vi "02_ui_smith_plot.vi"() -> ()   [LabVIEW 2025]
uses:
  213d4d69-42c2-4ab9-8e5c-f09799411473.vi
  9924c898-3be5-4834-b900-de0bc968c1de.vi
  9ab8033c-be5d-4a17-bbd5-1ebfae571c10.vi
panel:
  out "r_norm":dbl caption="Cursor - R"
  out "jx_norm":dbl caption="Cursor - jX"
  out "phase_cursor":dbl caption="Phase"
  out "jx_cursor":dbl caption="jX"
  out "r_cursor":dbl caption="R"
  out "smith_dimensions":i16
  out "frequency_cursor":string caption="Frequency"
  out "panel_resized":bool=TRUE
  out "smith_plot":picture
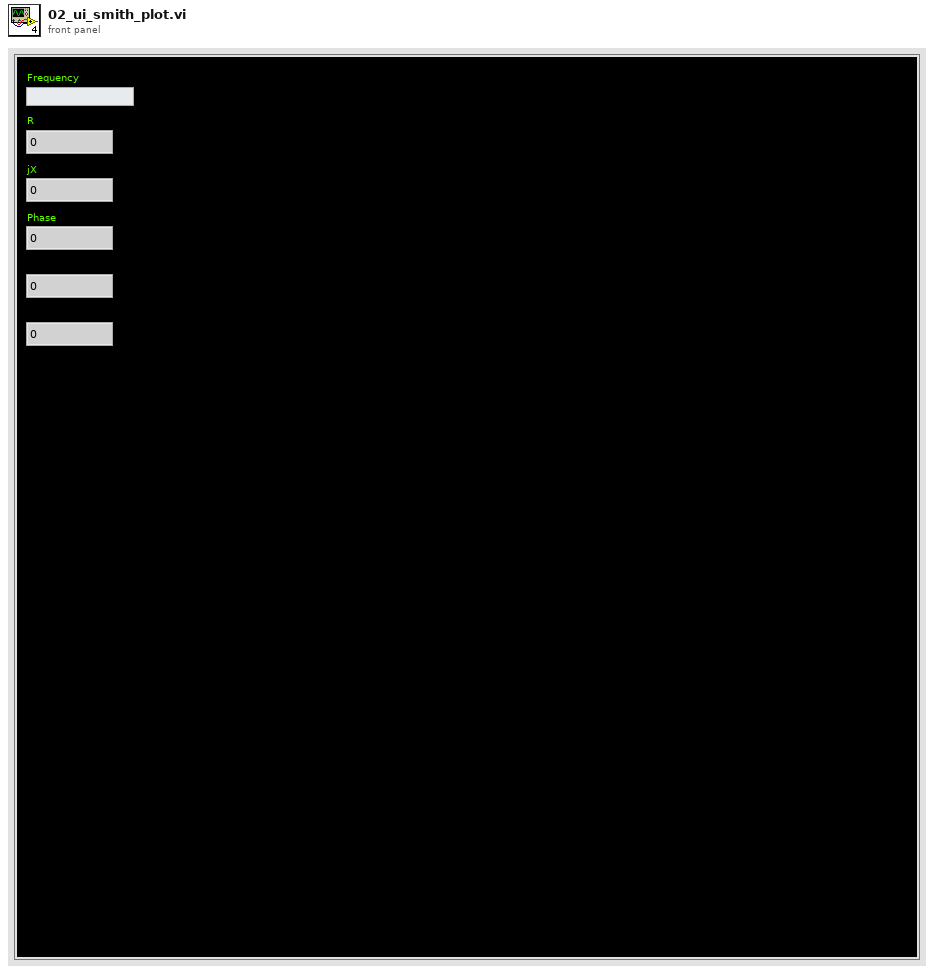
[diagram p1: front panel]
types:
  T1 = cluster{"button_load_sxp":bool, "button_load_csv":bool, "button_save_s1p":bool, "button_save_s2p":bool, "button_single_sweep":bool, "show_smith_window":bool}
  T2 = cluster{"freq_array":dbl[], "data_array":dbl[]}[]
  T3 = typedef "LVRectTypeDef.ctl" = cluster{"Left":i16, "Top":i16, "Right":i16, "Bottom":i16}
  T4 = typedef "LVPoint32TypeDef.ctl" = cluster{"Horizontal":i32, "Vertical":i32}
  T5 = cluster{"frequency":dbl, "r":dbl, "jx":dbl, "phase":dbl}
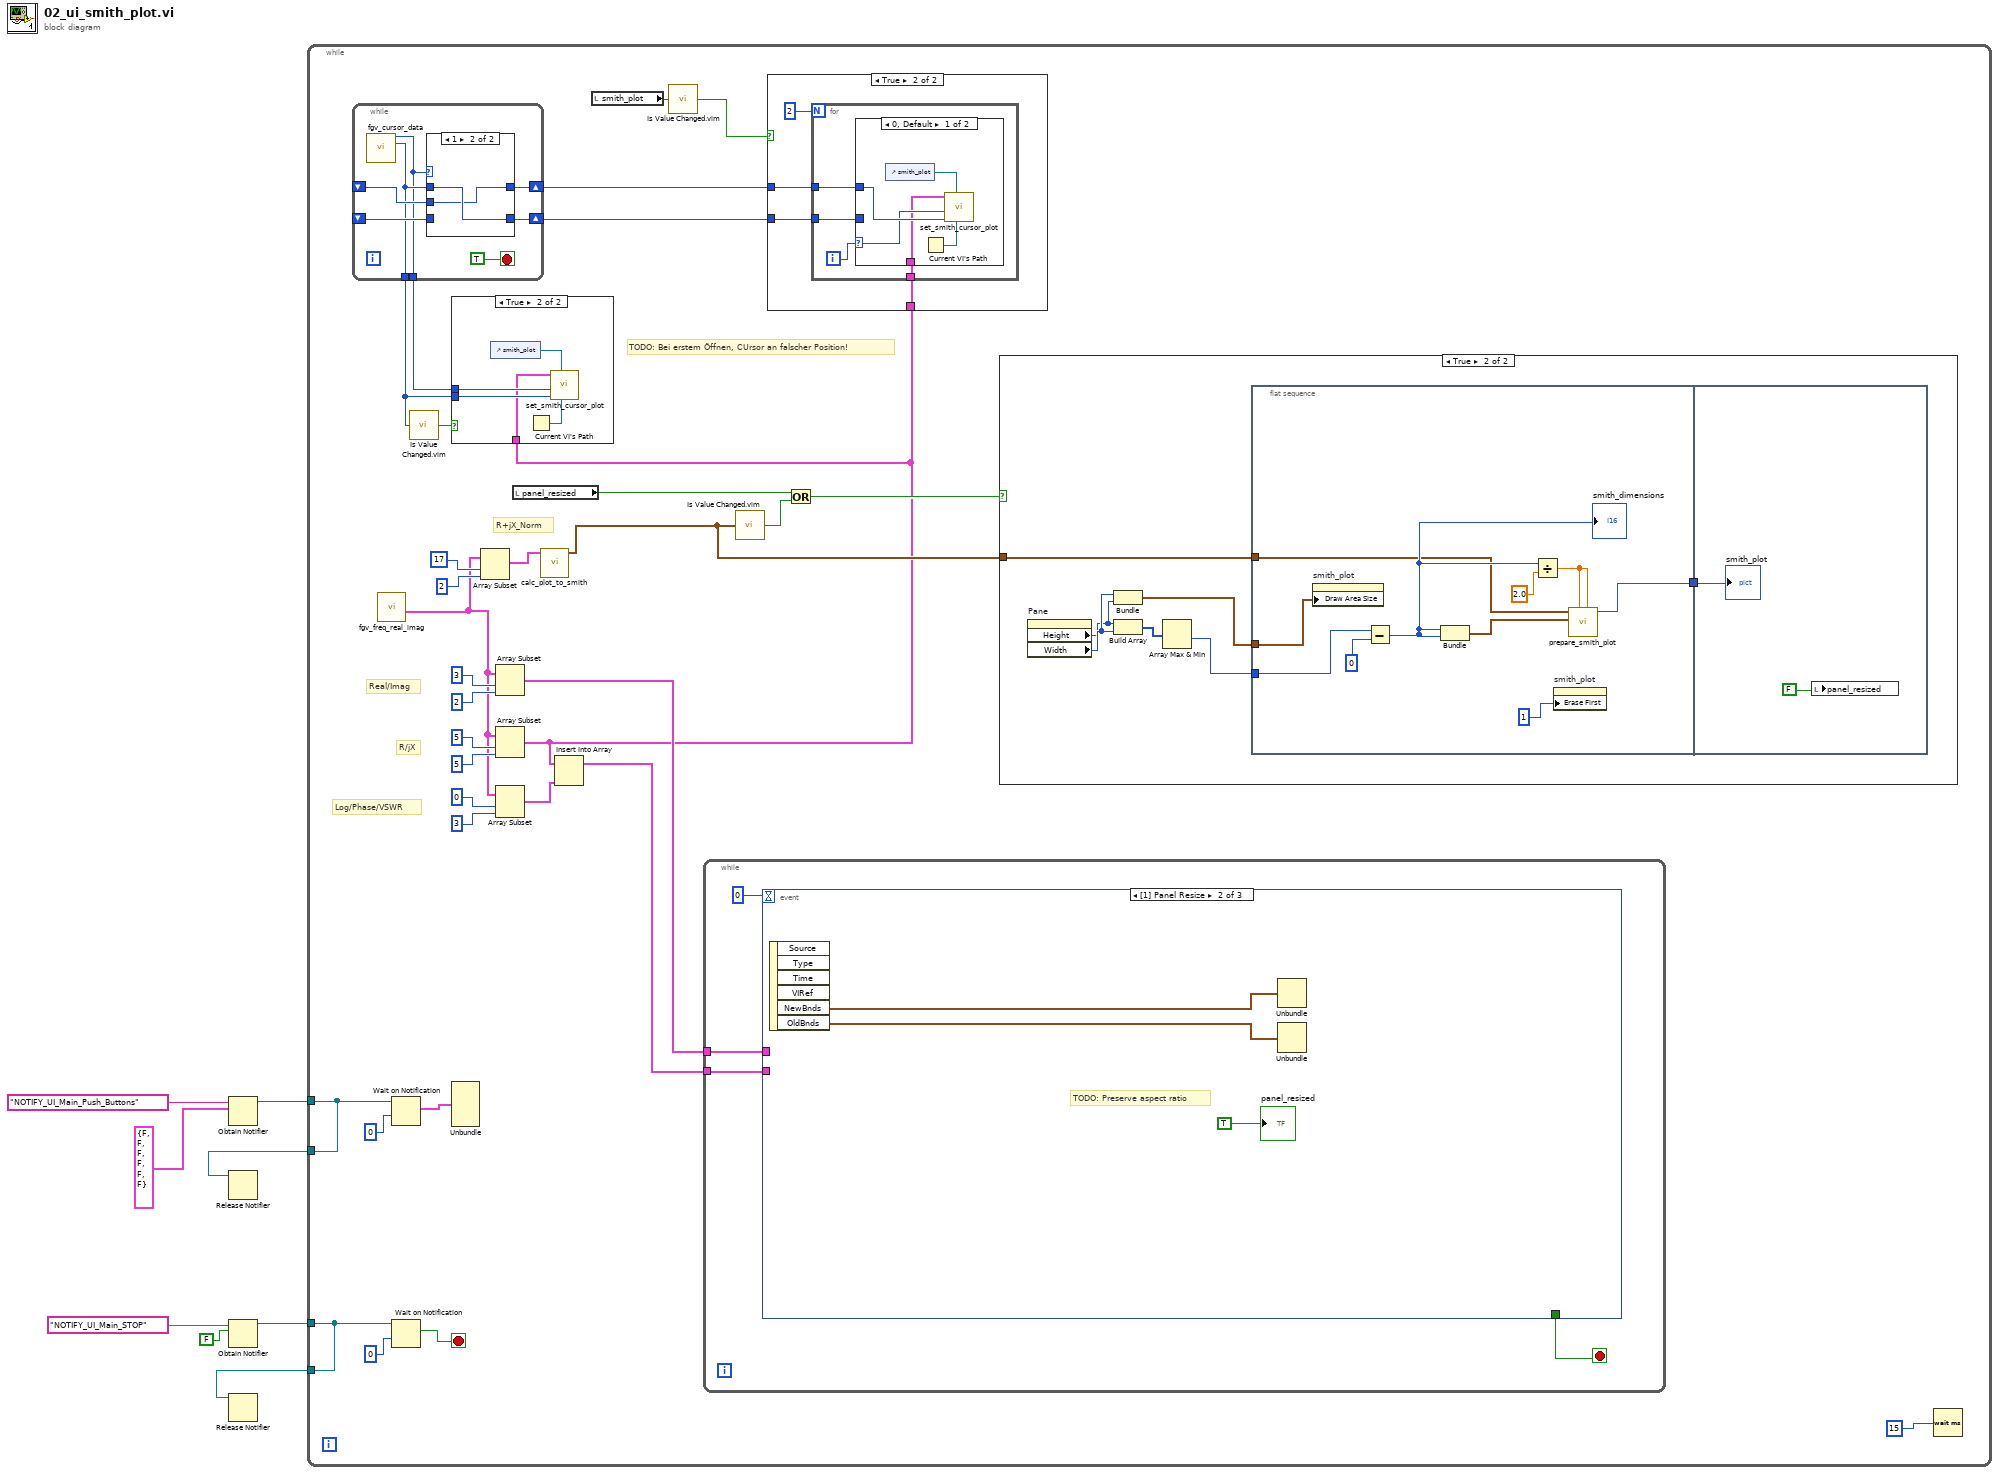
[diagram p0: block diagram]
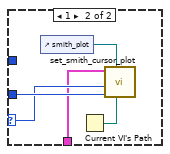
[diagram p4: hidden frame]
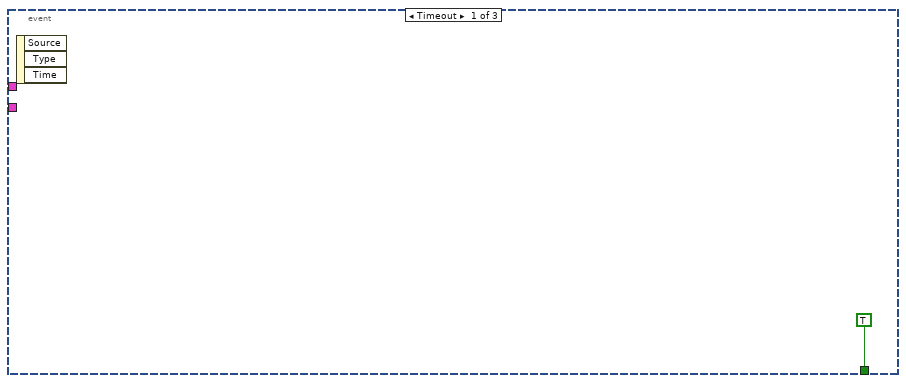
[diagram p6: hidden frame]
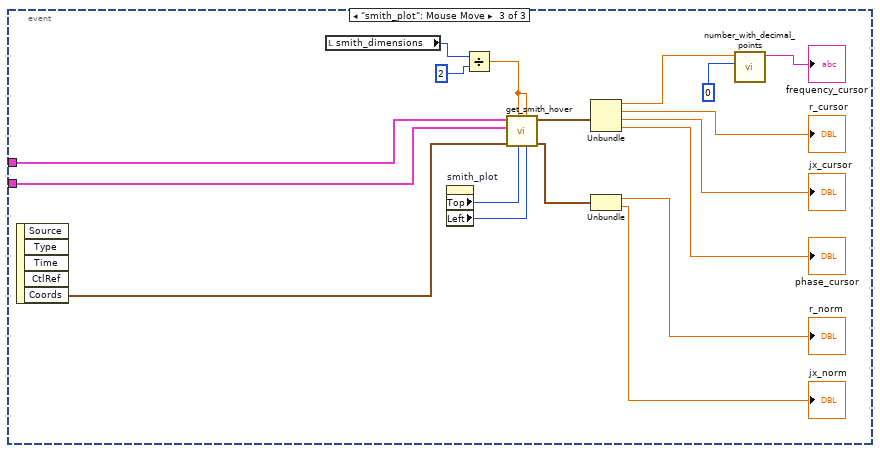
[diagram p7: hidden frame]
diagram:
  n1 = Obtain Notifier(name (unnamed)="NOTIFY_UI_Main_Push_Buttons", notification data type=T1 {"button_load_sxp"=FALSE, "button_load_csv"=FALSE, "button_save_s1p"=FALSE, "button_save_s2p"=FALSE, "button_single_sweep"=FALSE, "show_smith_window"=FALSE} ("output cluster")) -> (notifier out=w2:refnum<notifier>)  [unwired: 2 in, 2 out]
  n2 = Obtain Notifier(name (unnamed)="NOTIFY_UI_Main_STOP", notification data type=FALSE) -> (notifier out=w6:refnum<notifier>)  [unwired: 2 in, 2 out]
  n3 = while {
    tunnel: w6 -> [w36]
    tunnel: [w36] -> w5
    tunnel: w2 -> [w29]
    tunnel: [w29] -> w1
    stop <- w35 stop-if-true
    # "TODO: Bei erstem Öffnen, CUrsor an falscher Position!"
    # "Log/Phase/VSWR"
    # "R/jX"
    # "Real/Imag"
    # "R+jX_Norm"
    n4 = while {
      shift-right: [w69] -> w16
      shift-left: _ -> [w67]
      shift-right: [w68] -> w17
      shift-left: _ -> [w66]
      tunnel: [w65] -> w12
      tunnel: [w64] -> w15
      stop <- TRUE stop-if-true
      n5 = call "fgv_cursor_data.vi"() -> ("cursor_idx_get"=w64:i32, "cursor_pos_get"=w65:i32)  [unwired: 9 in, 5 out]
      n6 = case shown="1" w64 {
        tunnel: w65 -> [w72 w74]
        tunnel: [w72 w73] -> w69
        tunnel: [w71 w74] -> w68
        tunnel: w67 -> [_ w73]
        tunnel: w66 -> [w71 _]
        frame 0, Default {
        }
        frame 1 {
        }
      }
    }
    n7 = call "fgv_freq_real_imag.vi"() -> ("plot_data"=w18:T2)  [unwired: 8 in, 3 out]
    n8 = Wait on Notification(notifier=w29, timeout in ms (-1)=0) -> (notification=w31:T1)  [unwired: 2 in, 3 out]
    n9 = Wait on Notification(notifier=w36, timeout in ms (-1)=0) -> (notification=w35:bool)  [unwired: 2 in, 3 out]
    n10 = call "Is Value Changed.vim"("value"=w12) -> ("changed or first call?"=w11:bool)
    n11 = Unbundle(w31) -> ()  [unwired: 6 out]
    n12 = Array Subset(array=w18, index=17, length=2) -> (w32:T2)
    n13 = Array Subset(array=w18, index=3, length=2) -> (w20:T2)
    n14 = Array Subset(array=w18, index=5, length=5) -> (w14:T2)
    n15 = case shown="True" w11 {
      tunnel: w12 -> [_ w43]
      tunnel: w15 -> [_ w42]
      tunnel: w14 -> [_ w41]
      frame False {
      }
      frame True {
        n16 = control-ref of="smith_plot"() -> (w44:refnum<vi>)
        n17 = Current VI's Path() -> (path=w45:path)
        n18 = call "set_smith_cursor_plot.vi"("path"=w45, "smith_plot"=w44, "cursor_pos"=w43, "cursor_index"=w42, "plot_rjx"=w41) -> ()  [unwired: 7 in]
      }
    }
    n19 = Array Subset(array=w18, index=0, length=3) -> (w22:T2)
    n20 = local read "panel_resized"() -> (w10:bool)
    n21 = call "calc_plot_to_smith.vi"("Plot_Data"=w32) -> ("smith plot"=w19:cluster{"r":dbl, "x":dbl}[])  [unwired: 10 in]
    n22 = Insert Into Array(array=w14, new element=w22) -> (w21:T2)  [unwired: 1 in]
    n23 = local read "smith_plot"() -> (w13:picture)
    n24 = call "Is Value Changed.vim"("value"=w13) -> ("changed or first call?"=w9:bool)
    n25 = while {
      tunnel: w21 -> [w76]
      tunnel: w20 -> [w75]
      stop <- w77 stop-if-true
      n26 = event shown="[1] Panel Resize" {
        selector: _ -> [_ _ _]
        dyn-events: _ -> [_ _ _]
        timeout: 0 -> [_ _ _]
        tunnel: [TRUE _ _] -> w77
        tunnel: w76 -> [_ _ w84]
        tunnel: w75 -> [_ _ w83]
        event Timeout {
          n27 = event-data() -> ()  [unwired: 1 in, 3 out]
        }
        event Panel Resize {
          # "TODO: Preserve aspect ratio"
          n28 = event-data() -> ("NewBnds"=w80:T3, "OldBnds"=w81:T3)  [unwired: 1 in, 4 out]
          n29 = Unbundle(w80) -> ()  [unwired: 4 out]
          n30 = Unbundle(w81) -> ()  [unwired: 4 out]
          "panel_resized" <- TRUE
        }
        event "smith_plot": Mouse Move {
          n31 = event-data() -> ("Coords"=w100:T4)  [unwired: 1 in, 4 out]
          n32 = local read "smith_dimensions"() -> (w95:i16)
          n33 = property on="smith_plot" class="Pict"() -> ("Top"=w98:i32, "Left"=w97:i32)  [unwired: 2 in, 2 out]
          n34 = Divide(x=w95, y=u32 2) -> (x/y=w93:dbl)
          n35 = call "get_smith_hover.vi"("smith_pos_left"=w97, "left_center"=w93, "smith_pos_top"=w98, "top_center"=w93, "Coords"=w100, "cursor_data"=w84, "ref_data"=w83) -> ("cursor_pos"=w87:cluster{"r_norm":dbl, "x_norm":dbl}, "cursor_data"=w92:T5)  [unwired: 3 in]
          n36 = Unbundle(w92) -> ("frequency"=w88:dbl, "r"=→"r_cursor":dbl, "jx"=→"jx_cursor":dbl, "phase"=→"phase_cursor":dbl)
          n37 = Unbundle(w87) -> ("r_norm"=→"r_norm":dbl, "x_norm"=→"jx_norm":dbl)
          n38 = call "number_with_decimal_points.vi"("Precision"=i16 0, "Double"=w88) -> ("String"=→"frequency_cursor":string)  [unwired: 5 in]
        }
      }
    }
    n39 = call "Is Value Changed.vim"("value"=w19) -> ("changed or first call?"=w38:bool)
    n40 = case shown="True" w9 {
      tunnel: w16 -> [_ w48]
      tunnel: w17 -> [_ w47]
      tunnel: w14 -> [_ w46]
      frame False {
      }
      frame True {
        n41 = for {
          N: 2 -> [_]
          tunnel: w48 -> [w52]
          tunnel: w47 -> [w51]
          tunnel: w46 -> [w50]
          i -> [w53]
          n42 = case shown="0, Default" w53 {
            selector: w53 -> [w55 w60]
            tunnel: w52 -> [w56 _]
            tunnel: w51 -> [_ w61]
            tunnel: w50 -> [w54 w59]
            frame 0, Default {
              n43 = control-ref of="smith_plot"() -> (w58:refnum<vi>)
              n44 = Current VI's Path() -> (path=w57:path)
              n45 = call "set_smith_cursor_plot.vi"("path"=w57, "smith_plot"=w58, "cursor_pos"=w56, "cursor_index"=w55, "plot_rjx"=w54) -> ()  [unwired: 7 in]
            }
            frame 1 {
              n46 = control-ref of="smith_plot"() -> (w63:refnum<vi>)
              n47 = Current VI's Path() -> (path=w62:path)
              n48 = call "set_smith_cursor_plot.vi"("path"=w62, "smith_plot"=w63, "cursor_pos"=w61, "cursor_index"=w60, "plot_rjx"=w59) -> ()  [unwired: 7 in]
            }
          }
        }
      }
    }
    n49 = Or(x=w10, y=w38) -> (x .or. y?=w39:bool)
    n50 = case shown="True" w39 {
      tunnel: w19 -> [_ w102]
      frame False {
      }
      frame True {
        n51 = property on="Pane" class="Pane"() -> ("Height"=w105:u32, "Width"=w106:u32)  [unwired: 2 in, 2 out]
        n52 = Bundle("Width"=w106, "Height"=w105) -> (w104:cluster{"Width":u32, "Height":u32})  [unwired: 1 in]
        n53 = Build Array(w105, w106) -> (w107:u32[])
        n54 = Array Max & Min(array=w107) -> (min value=w101:u32)  [unwired: 3 out]
        n55 = flat-sequence {
          tunnel: w101 -> [w116]
          tunnel: w104 -> [w114]
          tunnel: [w109] -> w103
          tunnel: w102 -> [w108]
          tunnel: w103 -> [w118]
          frame #0 {
            n56 = property on="smith_plot" class="Pict"("Draw Area Size"=w114) -> ()  [unwired: 2 in, 2 out]
            n57 = Subtract(x=w116, y=u32 0) -> (x-y=w112:u32)
            "smith_dimensions" <- w112
            n58 = Bundle(w112, w112) -> (w111:cluster{u32, u32})  [unwired: 1 in]
            n59 = Divide(x=w112, y=2.0) -> (x/y=w110:dbl)
            n60 = property on="smith_plot" class="Pict"("Erase First"=u8 1) -> ()  [unwired: 2 in, 2 out]
            n61 = call "prepare_smith_plot.vi"("left_center"=w110, "top_center"=w110, "dimensions (w,h)"=w111, "smith plot"=w108) -> ("smith_out"=w109:picture)  [unwired: 7 in]
          }
          frame #1 {
            n62 = local write "panel_resized"(FALSE ("Boolean")) -> ()
            "smith_plot" <- w118
          }
        }
      }
    }
    n63 = Wait (ms)(milliseconds to wait=u32 15) -> ()  [unwired: 1 out]
  }
  n64 = Release Notifier(notifier=w1) -> ()  [unwired: 2 in, 3 out]
  n65 = Release Notifier(notifier=w5) -> ()  [unwired: 2 in, 3 out]
